vi "Agilent 2000 3000 X-Series Waveform Generator.vi"() -> ()   [LabVIEW 2015]
doc: "This example shows how to configure and output a user specific waveform. \n\n<B>Note:</B> This example is only applicable for the models which have the waveform generator license."
uses:
  Agilent 2000 3000 X-Series.lvlib
panel:
  in  "Enable Output (F: Disable)":bool
  in  "Offset (0.0 V)":dbl
  in  "Amplitude (1.0 V)":dbl=1.0
  in  "Frequency (1000 Hz)":dbl=1000.0
  in  "Function Type (0: Sine)":i32(ring) items=["Sine", "Square", "Ramp", "Pulse", "Noise", "DC"]
  in  "VISA resource name":refnum<visa-resource-name>
  # "(c) 2011-2023 National Instruments.  ALL RIGHTS RESERVED."
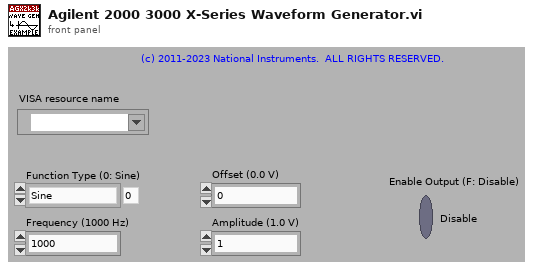
[diagram p1: front panel]
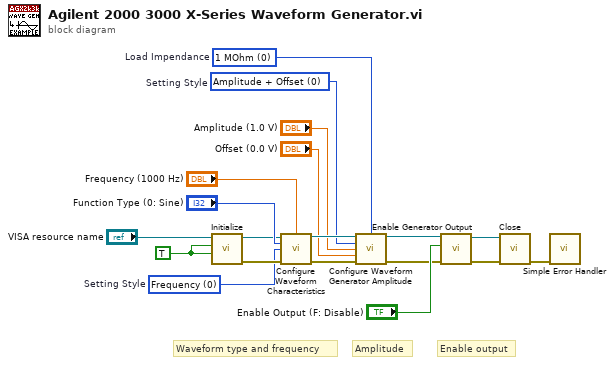
[diagram p0: block diagram]
diagram:
  w1 = 0 items=["1 MOhm", "50 Ohm"]  # Load Impendance
  w2 = 0 items=["Amplitude + Offset", "High Level + Low Level"]  # Setting Style
  w13 = 0 items=["Frequency", "Period"]  # Setting Style
  w18 = TRUE ("ID Query (True)")
  # "Enable output"
  # "Amplitude"
  # "Waveform type and frequency"
  n1 = call "Initialize.vi"("Reset (True)"=w18, "ID Query (True)"=w18, "VISA resource name"="VISA resource name") -> ("error out"=w15:errorcluster, "VISA resource name out"=w16:refnum<visa-resource-name>)  [unwired: 1 in, 6 out]
  n2 = call "Configure Waveform Characteristics.vi"("VISA resource name"=w16, "Frequency (1000 Hz)"="Frequency (1000 Hz)", "Function Type (0: Sine)"="Function Type (0: Sine)", "Setting Style (0: Frequency)"=w13, "error in (no error)"=w15) -> ("VISA resource name out"=w8:refnum<visa-resource-name>, "error out"=w6:errorcluster)  [unwired: 6 in, 3 out]
  n3 = call "Configure Waveform Generator Amplitude.vi"("VISA resource name"=w8, "Load Impedance (0: 1 MOhm)"=w1, "Setting Style (0: Amplitude + Offset)"=w2, "Amplitude (1.0 V)"="Amplitude (1.0 V)", "Offset (0.0 V)"="Offset (0.0 V)", "error in (no error)"=w6) -> ("VISA resource name out"=w7:refnum<visa-resource-name>, "error out"=w5:errorcluster)  [unwired: 8 in]
  n4 = call "Enable Generator Output.vi"("error in (no error)"=w5, "Enable Output (F: Disable)"="Enable Output (F: Disable)", "VISA resource name"=w7) -> ("error out"=w10:errorcluster, "VISA resource name out"=w11:refnum<visa-resource-name>)  [unwired: 1 in, 6 out]
  n5 = call "Close.vi"("error in (no error)"=w10, "VISA resource name"=w11) -> ("error out"=w9:errorcluster)  [unwired: 9 out]
  n6 = call <vilib>:"Simple Error Handler.vi"("error in (no error)"=w9) -> ()  [unwired: 1 in, 8 out]
